vi "_Read CSM File Logger Configuration - v1.0.vi"(7 "Section Name":string="FileLogger", 8 "error in (no error)":errorcluster, 11 "LabVIEW-Config.lvlib:LabVIEW-Config.lvclass":refnum<class "LabVIEW-Config.lvclass">) -> (0 "error out":errorcluster, 1 "FileLogger Configuration-v1":T1={"Enable"=TRUE, "Limit"={"FileSize"=10000000, "FileNum"=2}, "Timestamp.Format"="%<%Y/%m/%d %H:%M:%S%3u>T", "AutoExit"=FALSE} {"Limit"."FileSize" format="%.0p"}, 3 "Config out":refnum<class "LabVIEW-Config.lvclass">)   [LabVIEW 2017, in "INI-Static-Variable-Support.lvlib"]
uses:
  INI-Static-Variable-Support.lvlib
  LabVIEW-Config/LabVIEW-Config.lvclass
  2363d8f5-854b-48a2-904c-6eae4ebb3799.vi
  f10eeff7-a862-4cba-aa8a-b7c4c7649f5c.vi
  29f3f01c-bffc-45cc-bee5-2c053988ee4f.vi
  82b5d8dd-0cf4-4e1f-a111-323d7a64f2e5.vi
  <userlib>/_NEVSTOP/Communicable State Machine(CSM)/addons/API-String-Arugments-Support/_Support/Convert API String Arguments to Data(variant).vi
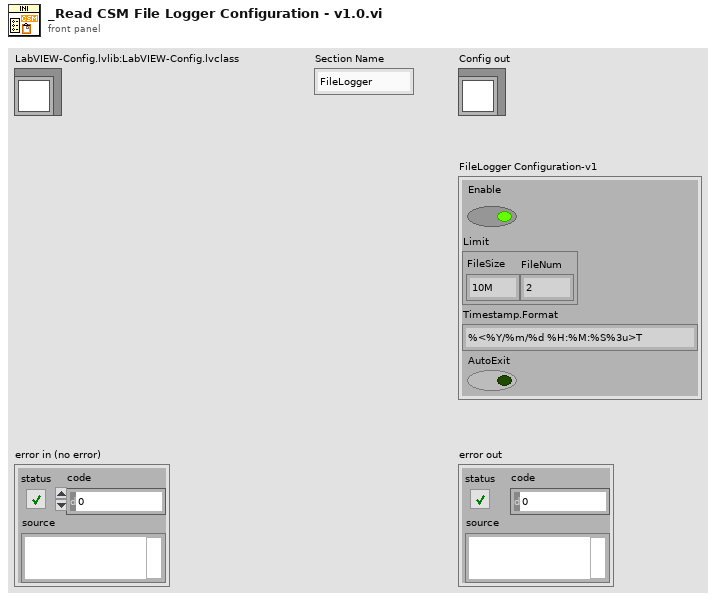
[diagram p1: front panel]
types:
  T1 = cluster{"Enable":bool, "Limit":cluster{"FileSize":i64, "FileNum":i32}, "Timestamp.Format":string, "AutoExit":bool}
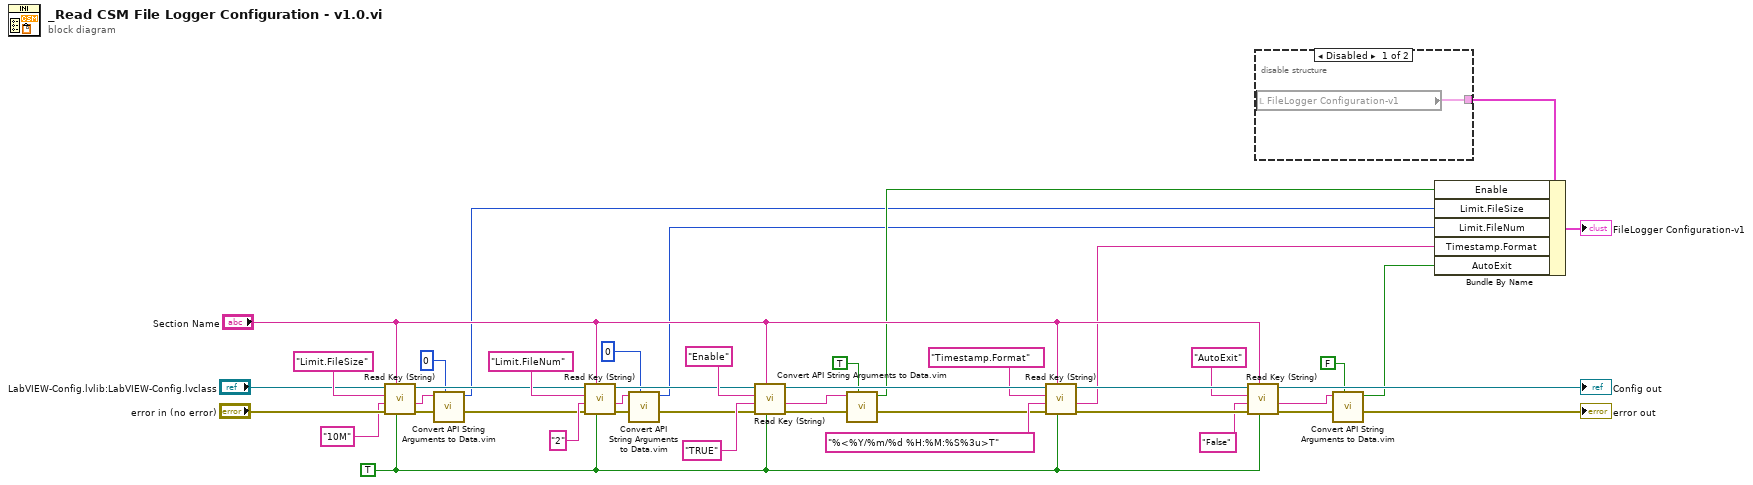
[diagram p0: block diagram]
diagram:
  w1 = TRUE ("Read Raw String? (F)")
  n1 = call "Read Key (String).vi"("Read Raw String? (F)"=w1, "Section Name"="Section Name", "error in (no error)"="error in (no error)", "Default"="10M", "Key Name"="Limit.FileSize", "Config in"="LabVIEW-Config.lvlib:LabVIEW-Config.lvclass") -> ("error out"=w29:errorcluster, "Value"=w13:string, "Config out"=w28:refnum<class "LabVIEW-Config.lvclass">)  [unwired: 2 in, 1 out]
  n2 = call "Convert API String Arguments to Data.vim"("Type"=i64 0 ("Limit.FileSize"), "error in (no error)"=w29, "String"=w13) -> ("error"=w16:errorcluster, "Data"=w4:i64)  [unwired: 5 in]
  n3 = call "Read Key (String).vi"("Read Raw String? (F)"=w1, "Section Name"="Section Name", "error in (no error)"=w16, "Default"="2", "Key Name"="Limit.FileNum", "Config in"=w28) -> ("error out"=w26:errorcluster, "Value"=w12:string, "Config out"=w27:refnum<class "LabVIEW-Config.lvclass">)  [unwired: 2 in, 1 out]
  n4 = call "Convert API String Arguments to Data.vim"("Type"=0 ("Limit.FileNum"), "error in (no error)"=w26, "String"=w12) -> ("error"=w17:errorcluster, "Data"=w2:i32)  [unwired: 5 in]
  n5 = call "Read Key (String).vi"("Read Raw String? (F)"=w1, "Section Name"="Section Name", "error in (no error)"=w17, "Default"="TRUE", "Key Name"="Enable", "Config in"=w27) -> ("error out"=w37:errorcluster, "Value"=w11:string, "Config out"=w38:refnum<class "LabVIEW-Config.lvclass">)  [unwired: 2 in, 1 out]
  n6 = call "Convert API String Arguments to Data.vim"("Type"=TRUE, "error in (no error)"=w37, "String"=w11) -> ("error"=w15:errorcluster, "Data"=w8:bool)  [unwired: 5 in]
  n7 = call "Read Key (String).vi"("Read Raw String? (F)"=w1, "Section Name"="Section Name", "error in (no error)"=w15, "Default"="%<%Y/%m/%d %H:%M:%S%3u>T", "Key Name"="Timestamp.Format", "Config in"=w38) -> ("error out"=w40:errorcluster, "Value"=w24:string, "Config out"=w41:refnum<class "LabVIEW-Config.lvclass">)  [unwired: 2 in, 1 out]
  n8 = call "Read Key (String).vi"("Read Raw String? (F)"=w1, "Section Name"="Section Name", "error in (no error)"=w40, "Default"="False", "Key Name"="AutoExit", "Config in"=w41) -> ("error out"=w43:errorcluster, "Value"=w10:string, "Config out"=→"Config out":refnum<class "LabVIEW-Config.lvclass">)  [unwired: 2 in, 1 out]
  n9 = disable-structure "Diagram Disable Structure" shown="Disabled" {
    disable-tunnel: [w44 _] -> w34
    frame Disabled {
      n10 = local read "FileLogger Configuration-v1"() -> (w44:T1)
    }
    frame Enabled {
    }
  }
  n11 = call "Convert API String Arguments to Data.vim"("Type"=FALSE, "error in (no error)"=w43, "String"=w10) -> ("error"=→"error out":errorcluster, "Data"=w6:bool)  [unwired: 5 in]
  n12 = Bundle By Name(cluster=w34, "Enable"=w8, "Limit.FileSize"=w4, "Limit.FileNum"=w2, "Timestamp.Format"=w24, "AutoExit"=w6) -> (→"FileLogger Configuration-v1":T1)
